vi "Periodic Tasks.vi"(8 "error in":errorcluster) -> ()   [LabVIEW 2016]
doc: "This VI runs in parallel to other tasks. It can contain as many user-defined periodic loops as you need. These can carry out PID or other sorts of timed response."
uses:
  <vilib>/Instr/_visa.llb/VISA Configure Serial Port (Instr).vi
  FRC SimulatedRSC/Positions.vi
panel:
  out "read buffer":string
  in  "Search_Params":string[](array[string])=["x1", "y1", "z1", "x2", "y2", "z2"]
  out "Last Complete Message":string
  out "length":i32
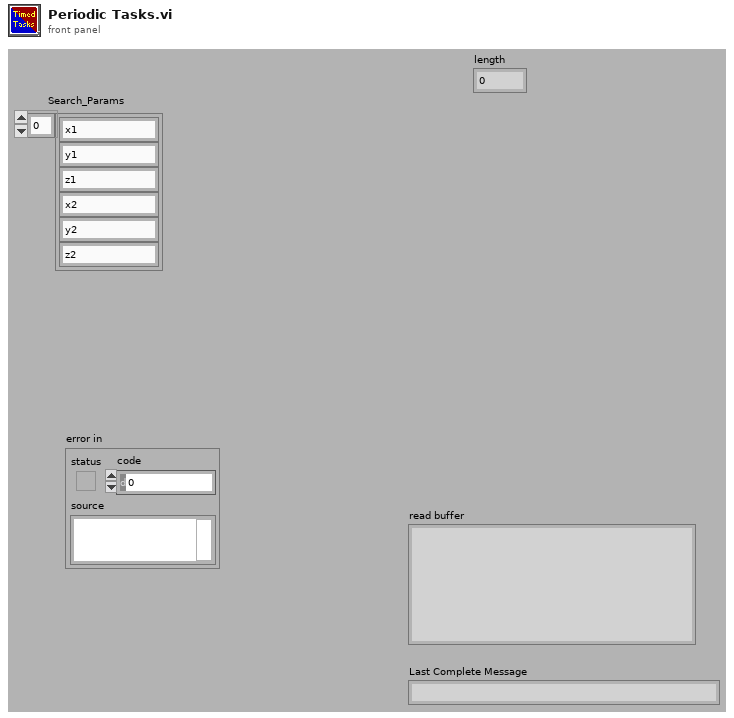
[diagram p1: front panel]
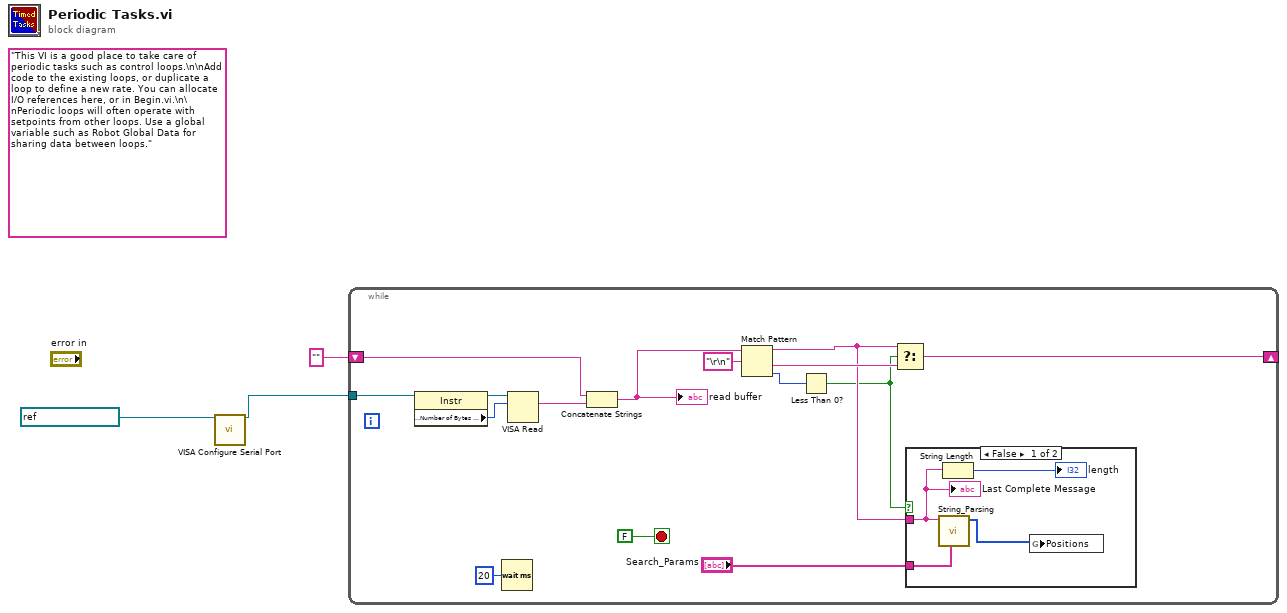
[diagram p0: block diagram]
diagram:
  (unwired) "This VI is a good place to take care of periodic tasks such as control loops.\n\nAdd code to the existing loops, or duplicate a loop to define a new rate. You can allocate I/O references here, or in Begin.vi.\n\nPeriodic loops will often operate with setpoints from other loops. Use a global variable such as Robot Global Data for sharing data between loops."
  n1 = call-poly "VISA Configure Serial Port"("VISA resource name"=refnum<visa-resource-name> "ASRL2::INSTR") -> ("VISA resource name out"=w2:refnum<visa-resource-name>)  [unwired: 13 in, 1 out]
  n2 = while {
    tunnel: w2 -> [w13]
    shift-right: [w5] -> _
    shift-left: "" -> [w12]
    stop <- FALSE stop-if-true
    n3 = property class="Instr"(reference=w13) -> (reference out=w17:refnum<visa-resource-name>, "Serial Settings:Number of Bytes at Serial Port"=w16:u32)  [unwired: 1 in, 1 out]
    n4 = Wait (ms)(milliseconds to wait=u32 20) -> ()  [unwired: 1 out]
    n5 = VISA Read(VISA resource name=w17, byte count=w16) -> (read buffer=w11:string)  [unwired: 1 in, 3 out]
    n6 = Concatenate Strings(w12, w11) -> (w10:string)
    "read buffer" <- w10
    n7 = Match Pattern(string=w10, regular expression="\r\n") -> (before substring=w6:string, after substring=w7:string, offset past match=w8:i32)  [unwired: 1 in, 1 out]
    n8 = Less Than 0?(x=w8) -> (x < 0?=w4:bool)
    n9 = Select(t=w6, s=w4, f=w7) -> (s? t:f=w5:string)
    n10 = case shown="False" w4 {
      tunnel: "Search_Params" -> [w22 _]
      tunnel: w6 -> [w21 _]
      frame False {
        n11 = call "String_Parsing.vi"("Search_Params"=w22, "Input"=w21) -> ("Positions"=w19:i32[])  [unwired: 9 in]
        n12 = String Length(string=w21) -> (length=→"length":i32)
        n13 = global write "Positions.vi" "Positions"(w19) -> ()
        "Last Complete Message" <- w21
      }
      frame True {
      }
    }
  }
